vi "USBcam_save.vi"() -> ()   [LabVIEW 2018]
uses:
  <vilib>/userdefined/High Color/IMAQdx.ctl
  <vilib>/vision/driver/IMAQdx.llb/IMAQdx Buffer Number Mode.ctl
  <vilib>/vision/driver/NI_Vision_Acquisition_Software.lvlib
panel:
  in  "Max rate (Hz)":i32=5
  in  "Measurement period (min)":dbl
  in  "Sampling rate (Hz)":i32=5
  out "Time stamp":path
  out "Movie file":path
  in  "Buffer Number Mode (Next)":T1
  in  "error constant":errorcluster
  in  "stop":bool
  in  "USB camera":T2
  out "Image":T3(plugin-control)
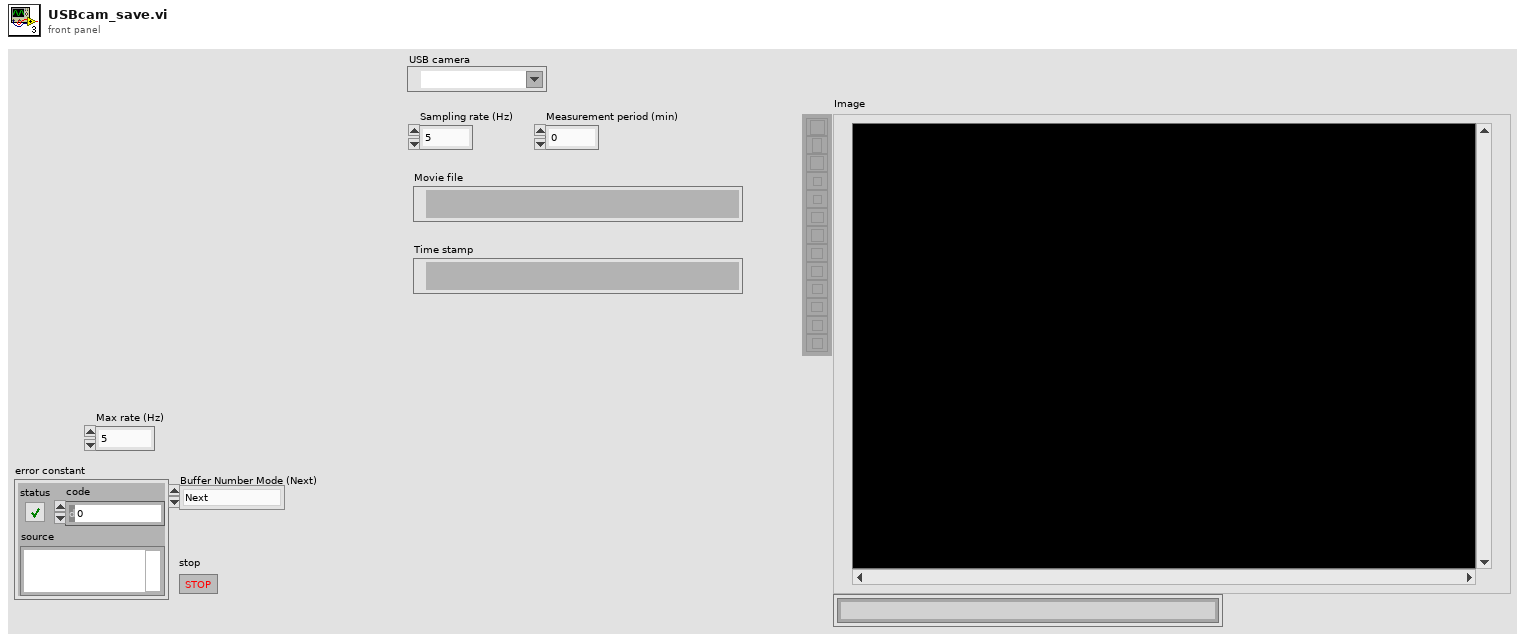
[diagram p1: front panel]
types:
  T1 = typedef "NI_Vision_Acquisition_Software.lvlib/IMAQdx Buffer Number Mode.ctl" = enum32{"Next", "Last", "Buffer Number", "Every", "Last New"}
  T2 = typedef "IMAQdx.ctl" = refnum<k21>
  T3 = typedef "IMAQ Image.ctl" = refnum<image>
  T4 = typedef "AviRefnum.ctl" = refnum<k1>
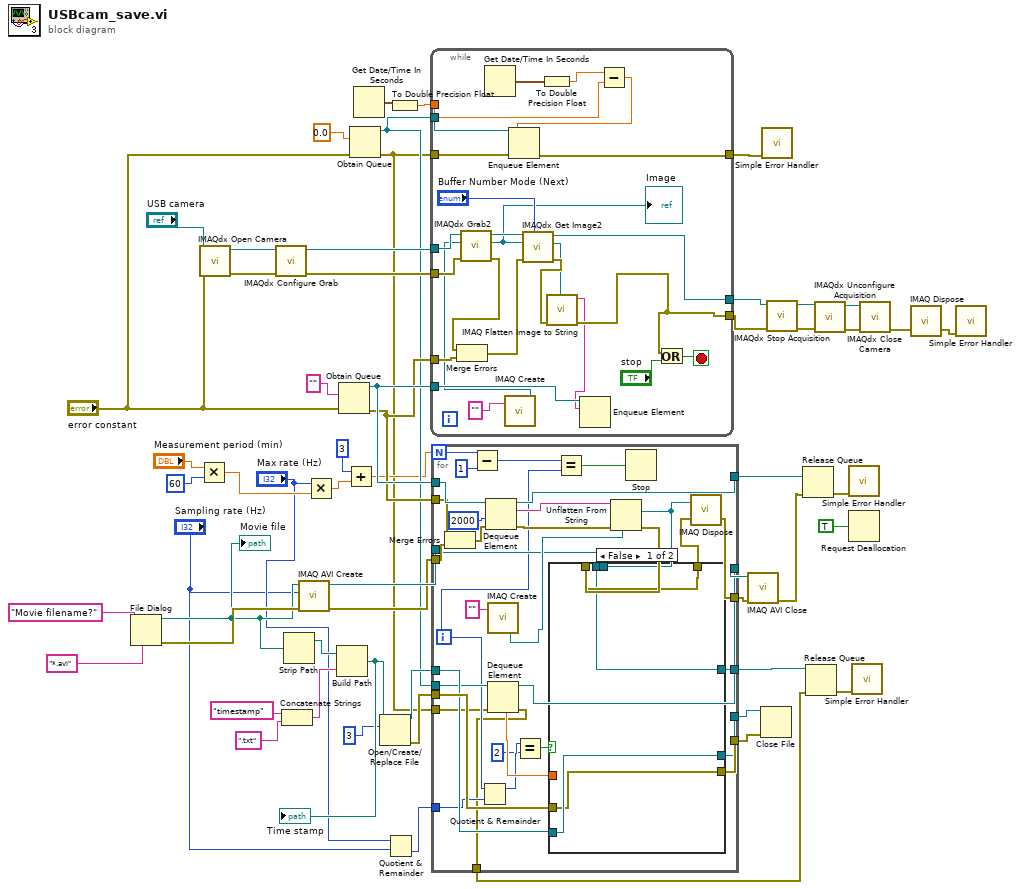
[diagram p0: block diagram]
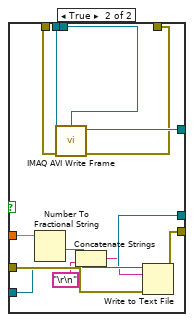
[diagram p2: hidden frame]
diagram:
  n1 = File Dialog(6:"*.avi" ("pattern"), 9:"Movie filename?" ("prompt")) -> (0:w32:errorcluster, 3:w27:path)  [unwired: 2 in, 5 out]
  "Movie file" <- w27
  n2 = Multiply(x="Measurement period (min)", y=60 ("timeout in ms (-1)")) -> (x*y=w9:dbl)
  n3 = call <vilib>:"IMAQdx Open Camera.vi"("error in"="error constant", "Session In"="USB camera") -> ("error out"=w55:errorcluster, "Session Out"=w56:T2)  [unwired: 8 in]
  n4 = call <vilib>:"IMAQdx Configure Grab.vi"("error in"=w55, "Session In"=w56) -> ("error out"=w43:errorcluster, "Session Out"=w45:T2)  [unwired: 8 in]
  n5 = Concatenate Strings("timestamp", ".txt" ("string")) -> (w28:string)
  n6 = Strip Path(path=w27) -> (stripped path=w29:path)  [unwired: 1 out]
  n7 = call "IMAQ AVI Create"("error in (no error)"=w32, "Frames Per Second"="Sampling rate (Hz)", "AVI Path"=w27) -> ("error out"=w39:errorcluster, "Avi Refnum"=w40:T4)  [unwired: 4 in, 3 out]
  n8 = Multiply(x="Max rate (Hz)", y=w9) -> (x*y=w8:dbl)
  n9 = Build Path(base path=w29, name or relative path=w28) -> (appended path=w26:path)
  "Time stamp" <- w26
  n10 = Obtain Queue(element data type="", error in (no error)="error constant") -> (queue out=w47:refnum<queue>, error out=w46:errorcluster)  [unwired: 3 in, 1 out]
  n11 = Add(x=3 ("timeout in ms (-1)"), y=w8) -> (x+y=w6:dbl)
  n12 = Obtain Queue(element data type=0.0, error in (no error)="error constant") -> (queue out=w12:refnum<queue>, error out=w2:errorcluster)  [unwired: 3 in, 1 out]
  n13 = Get Date/Time In Seconds() -> (seconds since 1Jan1904=w17:timestamp)
  n14 = Open/Create/Replace File(file path (use dialog)=w26, operation (0:open)=3 ("timeout in ms (-1)")) -> (refnum out=w24:refnum<file>, error out=w25:errorcluster)  [unwired: 4 in, 1 out]
  n15 = Quotient & Remainder(x="Max rate (Hz)", y="Sampling rate (Hz)") -> (floor(x/y)=w3:i32)  [unwired: 1 out]
  n16 = To Double Precision Float(number=w17) -> (double precision float=w16:dbl)
  n17 = while {
    tunnel: [w71] -> w48
    tunnel: w47 -> [w81]
    tunnel: w46 -> [w80]
    tunnel: w45 -> [w73]
    tunnel: [w74] -> w44
    tunnel: w43 -> [w78]
    tunnel: w16 -> [w63]
    tunnel: w12 -> [w61]
    tunnel: w2 -> [w59]
    tunnel: [w58] -> w13
    stop <- w65 stop-if-true
    n18 = Get Date/Time In Seconds() -> (seconds since 1Jan1904=w64:timestamp)
    n19 = call "IMAQ Create"("Image Name"="") -> ("New Image"=w72:T3)  [unwired: 4 in, 1 out]
    n20 = call <vilib>:"IMAQdx Grab2.vi"("error in"=w78, "Image In"=w72, "Session In"=w73) -> ("error out"=w77:errorcluster, "Image Out"=w66:T3, "Session Out"=w79:T2)  [unwired: 5 in, 1 out]
    "Image" <- w66
    n21 = Merge Errors(w77, w80) -> (w76:errorcluster)
    n22 = call <vilib>:"IMAQdx Get Image2.vi"("Buffer Number Mode (Next)"="Buffer Number Mode (Next)", "error in"=w76, "Image In"=w66, "Session In"=w79) -> ("error out"=w69:errorcluster, "Image Out"=w67:T3, "Session Out"=w74:T2)  [unwired: 4 in, 1 out]
    n23 = To Double Precision Float(number=w64) -> (double precision float=w62:dbl)
    n24 = call "IMAQ Flatten Image to String"("error in (no error)"=w69, "Image"=w67) -> ("error out"=w71:errorcluster, "Data String"=w70:string)  [unwired: 8 in]
    n25 = Enqueue Element(queue=w81, element=w70) -> ()  [unwired: 2 in, 3 out]
    n26 = Subtract(x=w62, y=w63) -> (x-y=w60:dbl)
    n27 = Enqueue Element(queue=w61, element=w60, error in (no error)=w59) -> (error out=w58:errorcluster)  [unwired: 1 in, 2 out]
    n28 = Or(x=w71, y="stop") -> (x .or. y?=w65:bool)
  }
  n29 = for {
    N: w6 -> [w98]
    tunnel: w47 -> [w116]
    tunnel: w46 -> [w110]
    tunnel: [w115] -> w41
    tunnel: [w90] -> w38
    tunnel: w39 -> [w108]
    tunnel: w40 -> [w107]
    tunnel: [w105] -> w36
    tunnel: w25 -> [w104]
    tunnel: w24 -> [w103]
    tunnel: [w102] -> w23
    tunnel: [w101] -> w22
    tunnel: w12 -> [w95]
    tunnel: [w93] -> w10
    tunnel: w3 -> [w89]
    tunnel: w2 -> [w84]
    tunnel: [w83] -> w1
    i -> [w85]
    n30 = Merge Errors(w110, w108) -> (w109:errorcluster)
    n31 = Subtract(x=w98, y=1 ("timeout in ms (-1)")) -> (x-y=w97:i32)
    n32 = Quotient & Remainder(x=w85, y=w89) -> (x-y*floor(x/y)=w88:i32)  [unwired: 1 out]
    n33 = Dequeue Element(queue=w116, timeout in ms (-1)=2000, error in (no error)=w109) -> (queue out=w115:refnum<queue>, element=w113:string, error out=w112:errorcluster)  [unwired: 1 out]
    n34 = call "IMAQ Create"("Image Name"="") -> ("New Image"=w111:T3)  [unwired: 3 in, 2 out]
    n35 = Dequeue Element(queue=w95, error in (no error)=w84) -> (queue out=w93:refnum<queue>, element=w94:dbl, error out=w83:errorcluster)  [unwired: 1 in, 1 out]
    n36 = Equal?(x=w88, y=2 ("timeout in ms (-1)")) -> (x = y?=w86:bool)
    n37 = Equal?(x=w97, y=w85) -> (x = y?=w99:bool)
    n38 = Unflatten From String(type=w111, binary string=w113, error in (no error)=w112) -> (value=w100:T3, error out=w106:errorcluster)  [unwired: 2 in, 1 out]
    n39 = case shown="False" w86 {
      tunnel: w107 -> [w118 w133]
      tunnel: w106 -> [w120 w132]
      tunnel: [w118 w131] -> w105
      tunnel: w104 -> [w117 w130]
      tunnel: w103 -> [w119 w129]
      tunnel: [w117 w128] -> w102
      tunnel: [w119 w127] -> w101
      tunnel: w100 -> [_ w123]
      tunnel: w94 -> [_ w122]
      tunnel: [w120 w121] -> w91
      frame False {
      }
      frame True {
        n40 = Number To Fractional String(number=w122) -> (F-format string=w125:string)  [unwired: 3 in]
        n41 = call "IMAQ AVI Write Frame"("error in (no error)"=w132, "Image"=w123, "Avi Refnum"=w133) -> ("error out"=w121:errorcluster, "Avi Refnum (duplicate)"=w131:T4)  [unwired: 1 in, 6 out]
        n42 = Concatenate Strings(w125, "\r\n") -> (w124:string)
        n43 = Write to Text File(file (use dialog)=w129, text=w124, error in=w130) -> (refnum out=w127:refnum<file>, error out=w128:errorcluster)  [unwired: 1 in, 1 out]
      }
    }
    n44 = Stop(stop? (T)=w99) -> ()
    n45 = call "IMAQ Dispose"("Image"=w100, "error in (no error)"=w91) -> ("error out"=w90:errorcluster)  [unwired: 4 in]
  }
  n46 = call "IMAQ AVI Close"("error in (no error)"=w38, "Avi Refnum"=w36) -> ("error out"=w37:errorcluster)  [unwired: 9 out]
  n47 = Close File(refnum=w22, error in=w23) -> ()  [unwired: 2 out]
  n48 = call <vilib>:"Simple Error Handler.vi"("error in (no error)"=w13) -> ()  [unwired: 4 in, 5 out]
  n49 = call <vilib>:"IMAQdx Stop Acquisition.vi"("error in"=w48, "Session In"=w44) -> ("error out"=w54:errorcluster, "Session Out"=w53:T2)  [unwired: 8 in]
  n50 = Release Queue(queue=w41, error in (no error)=w37) -> (error out=w21:errorcluster)  [unwired: 1 in, 2 out]
  n51 = Release Queue(queue=w10, error in (no error)=w1) -> (error out=w11:errorcluster)  [unwired: 1 in, 2 out]
  n52 = call <vilib>:"IMAQdx Unconfigure Acquisition.vi"("error in"=w54, "Session In"=w53) -> ("error out"=w52:errorcluster, "Session Out"=w51:T2)  [unwired: 8 in]
  n53 = call <vilib>:"Simple Error Handler.vi"("error in (no error)"=w21) -> ()  [unwired: 4 in, 5 out]
  n54 = Request Deallocation(TRUE ("flag")) -> ()
  n55 = call <vilib>:"Simple Error Handler.vi"("error in (no error)"=w11) -> ()  [unwired: 4 in, 5 out]
  n56 = call <vilib>:"IMAQdx Close Camera.vi"("error in"=w52, "Session In"=w51) -> ("error out"=w50:errorcluster)  [unwired: 9 in]
  n57 = call "IMAQ Dispose"("error in (no error)"=w50) -> ("error out"=w49:errorcluster)  [unwired: 5 in]
  n58 = call <vilib>:"Simple Error Handler.vi"("error in (no error)"=w49) -> ()  [unwired: 4 in, 5 out]
